vi "addDataDBLArray.vi"(0 "U8ArrayBuilderAutoIndexing in":refnum<class "U8ArrayBuilderAutoIndexing.lvclass">, 5 "Data":dbl[](array[numeric]), 7 "Length":i32, 9 "OverrideSwapBytes":bool, 11 "error in (no error)":errorcluster) -> (4 "U8ArrayBuilderAutoIndexing out":refnum<class "U8ArrayBuilderAutoIndexing.lvclass">, 15 "error out":errorcluster)   [LabVIEW 2016, in "RTUtilities.lvlib" / "U8ArrayBuilderAutoIndexing.lvclass"]
uses:
  U8ArrayBuilderAutoIndexing.lvclass
  U8ArrayBuilderAutoIndexing.lvclass/U8ArrayBuilderAutoIndexing.ctl
  U8ArrayBuilderManualIndexing/U8ArrayBuilderManualIndexing.lvclass
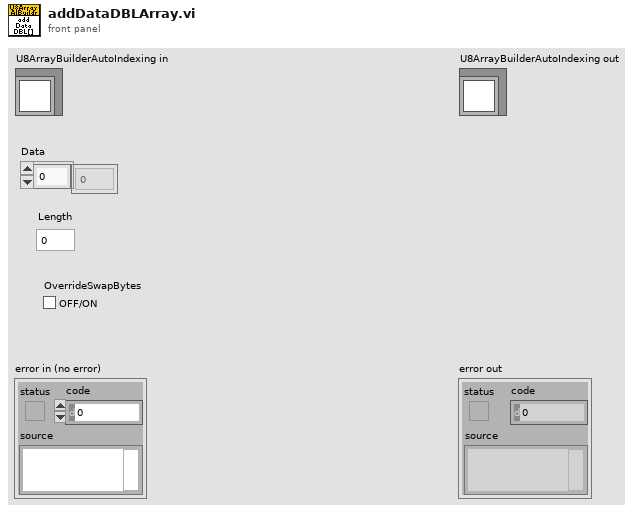
[diagram p1: front panel]
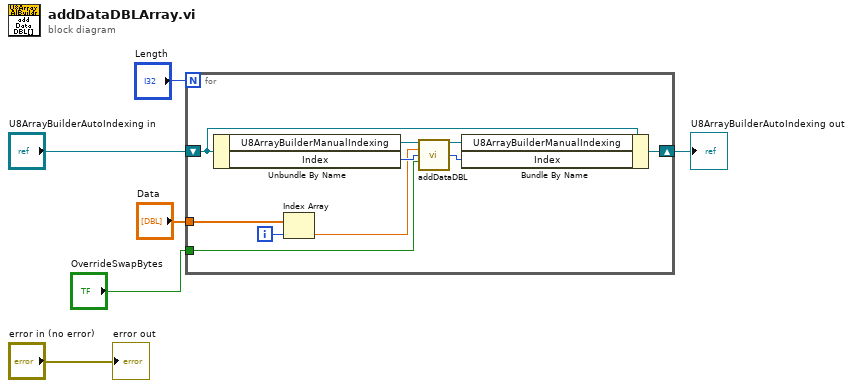
[diagram p0: block diagram]
diagram:
  n1 = for {
    N: "Length" -> [_]
    tunnel: "OverrideSwapBytes" -> [w13]
    shift-right: [w10] -> w3
    shift-left: "U8ArrayBuilderAutoIndexing in" -> [w16]
    tunnel: "Data" -> [w9]
    i -> [w8]
    n2 = Unbundle By Name(w16) -> ("U8ArrayBuilderManualIndexing"=w15:refnum<class "U8ArrayBuilderManualIndexing.lvclass">, "Index"=w14:i32)
    n3 = Index Array(array=w9, index=w8) -> (element=w7:dbl)
    n4 = call "addDataDBL.vi"("U8ArrayBuilderManualIndexing in"=w15, "Data"=w7, "Index"=w14, "OverrideSwapBytes"=w13) -> ("U8ArrayBuilderManualIndexing out"=w11:refnum<class "U8ArrayBuilderManualIndexing.lvclass">, "Index out"=w12:i32)  [unwired: 9 in, 1 out]
    n5 = Bundle By Name(cluster=w16, "U8ArrayBuilderManualIndexing"=w11, "Index"=w12) -> (w10:refnum<class "U8ArrayBuilderAutoIndexing.lvclass">)
  }
  "U8ArrayBuilderAutoIndexing out" <- w3
  "error out" <- "error in (no error)"
